vi "xcorr_packet bkp energy.vi"(0 "x":u32, 1 "y":u32, 2 "trigger":bool, 3 "normalization":u16) -> (8 "out":u64, 9 "valid":bool)   [LabVIEW 2017]
uses:
  <vilib>/rvi/FXPMathLib/FxpDiv/subVIs/nifxpmath_Div_SimConfig.ctl
  <vilib>/rvi/FXPMathLib/FxpDiv/simVIs/DllFxpDivTemp_sub.vi
  <vilib>/rvi/FXPMathLib/basic elements/FxpDiscreteDelay/XNode/nifxpmath_DiscreteDelay.xnode
  <vilib>/rvi/FXPMathLib/FxpMul/XNode/nifxpmath_Multiplier.xnode
  <vilib>/rvi/FXPMathLib/FxpDiv/XNode/nifxpmath_Div.xnode
  <vilib>/rvi/FXPMathLib/sim/FxpSim.dll
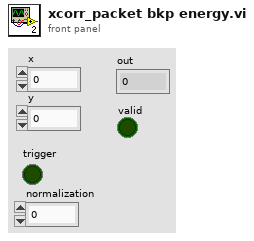
[diagram p1: front panel]
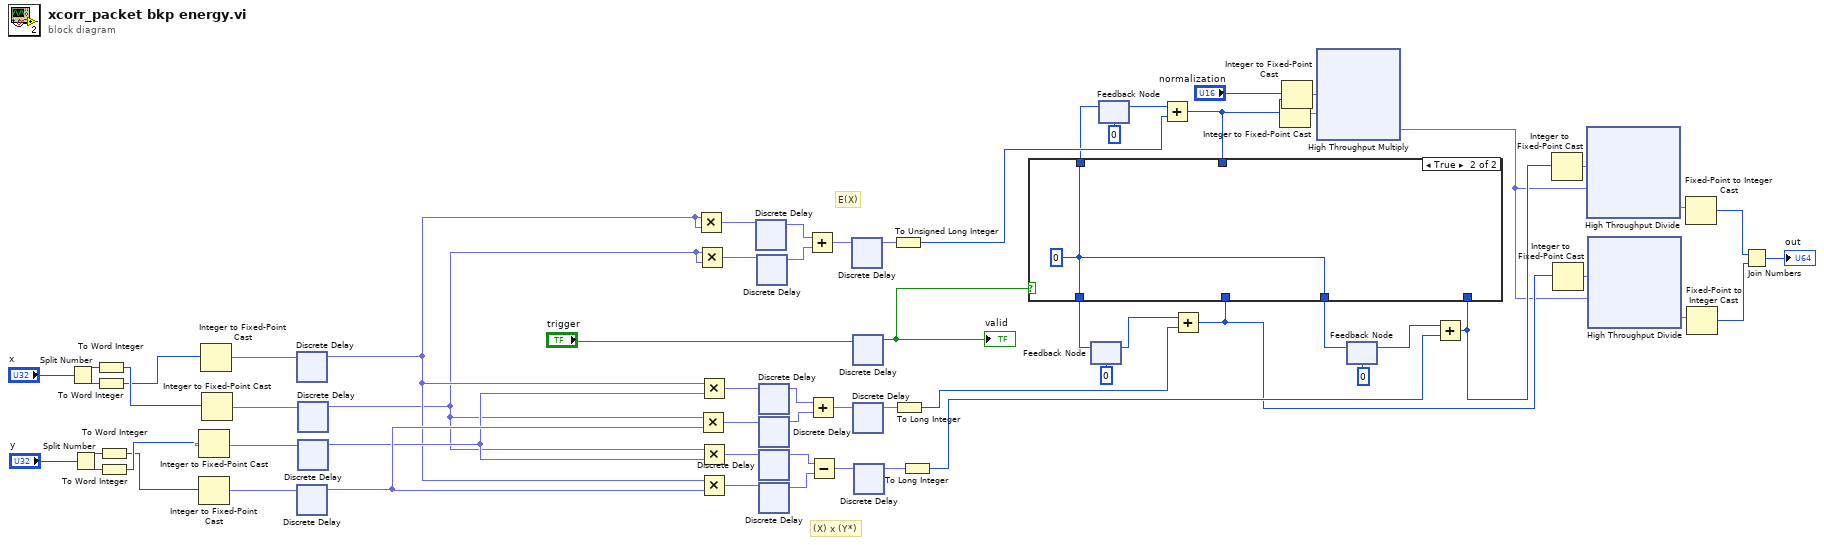
[diagram p0: block diagram]
diagram:
  # "E(X)"
  # "(X) x (Y*)"
  n1 = Split Number(x="x") -> (hi(x)=w55:u16, lo(x)=w56:u16)
  n2 = Split Number(x="y") -> (hi(x)=w57:u16, lo(x)=w58:u16)
  n3 = To Word Integer(number=w55) -> (16bit integer=w29:i16)
  n4 = To Word Integer(number=w56) -> (16bit integer=w28:i16)
  n5 = To Word Integer(number=w57) -> (16bit integer=w26:i16)
  n6 = To Word Integer(number=w58) -> (16bit integer=w27:i16)
  n7 = Integer to Fixed-Point Cast(integer=w27) -> (fixed-point=w38:fxp<+/-,16,16>)  [unwired: 1 in]
  n8 = Integer to Fixed-Point Cast(integer=w26) -> (fixed-point=w40:fxp<+/-,16,16>)  [unwired: 1 in]
  n9 = Integer to Fixed-Point Cast(integer=w28) -> (fixed-point=w36:fxp<+/-,16,16>)  [unwired: 1 in]
  n10 = Integer to Fixed-Point Cast(integer=w29) -> (fixed-point=w37:fxp<+/-,16,16>)  [unwired: 1 in]
  n11 = xnode "Discrete Delay"("D"=w36) -> ("Q"=w24:fxp<+/-,16,16>)
  n12 = xnode "Discrete Delay"("D"=w40) -> ("Q"=w39:fxp<+/-,16,16>)
  n13 = xnode "Discrete Delay"("D"=w37) -> ("Q"=w22:fxp<+/-,16,16>)
  n14 = xnode "Discrete Delay"("D"=w38) -> ("Q"=w34:fxp<+/-,16,16>)
  n15 = Multiply(x=w24, y=w24) -> (x*y=w25:fxp<+/-,32,32>)
  n16 = Multiply(x=w22, y=w22) -> (x*y=w23:fxp<+/-,32,32>)
  n17 = Multiply(x=w22, y=w39) -> (x*y=w46:fxp<+/-,32,32>)
  n18 = Multiply(x=w24, y=w34) -> (x*y=w45:fxp<+/-,32,32>)
  n19 = Multiply(x=w22, y=w34) -> (x*y=w47:fxp<+/-,32,32>)
  n20 = Multiply(x=w24, y=w39) -> (x*y=w48:fxp<+/-,32,32>)
  n21 = xnode "Discrete Delay"("D"=w25) -> ("Q"=w19:fxp<+/-,32,32>)
  n22 = xnode "Discrete Delay"("D"=w23) -> ("Q"=w18:fxp<+/-,32,32>)
  n23 = xnode "Discrete Delay"("D"=w45) -> ("Q"=w41:fxp<+/-,32,32>)
  n24 = xnode "Discrete Delay"("D"=w46) -> ("Q"=w42:fxp<+/-,32,32>)
  n25 = xnode "Discrete Delay"("D"=w47) -> ("Q"=w43:fxp<+/-,32,32>)
  n26 = xnode "Discrete Delay"("D"=w48) -> ("Q"=w44:fxp<+/-,32,32>)
  n27 = Add(x=w19, y=w18) -> (x+y=w20:fxp<+/-,33,33>)
  n28 = Add(x=w41, y=w42) -> (x+y=w51:fxp<+/-,33,33>)
  n29 = Subtract(x=w43, y=w44) -> (x-y=w50:fxp<+/-,32,32>)
  n30 = xnode "Discrete Delay"("D"=w20) -> ("Q"=w21:fxp<+/-,33,33>)
  n31 = xnode "Discrete Delay"("D"="trigger") -> ("Q"=w52:bool)
  "valid" <- w52
  n32 = xnode "Discrete Delay"("D"=w51) -> ("Q"=w35:fxp<+/-,33,33>)
  n33 = xnode "Discrete Delay"("D"=w50) -> ("Q"=w49:fxp<+/-,32,32>)
  n34 = To Unsigned Long Integer(number=w21) -> (unsigned 32bit integer=w15:u32)
  n35 = To Long Integer(number=w35) -> (32bit integer=w53:i32)
  n36 = To Long Integer(number=w49) -> (32bit integer=w54:i32)
  n37 = feedback #1(0) -> (w61:i32)
  n38 = feedback #2(0) -> (w16:u32)
  n39 = Add(x=w16, y=w15) -> (x+y=w2:u32)
  n40 = Add(x=w61, y=w53) -> (x+y=w8:i32)
  n41 = Integer to Fixed-Point Cast(integer=w2) -> (fixed-point=w3:fxp<+,32,32>)  [unwired: 1 in]
  n42 = Integer to Fixed-Point Cast(integer="normalization") -> (fixed-point=w4:fxp<+,16,16>)  [unwired: 1 in]
  n43 = xnode ("High Throughput Multiply")("x"=w4, "y"=w3) -> ("x*y"=w1:fxp<+,48,48>)
  n44 = feedback #3(0) -> (w31:i32)
  n45 = Add(x=w31, y=w54) -> (x+y=w9:i32)
  n46 = case shown="True" w52 {
    tunnel: [w67 w68] -> w32
    tunnel: [w66 w68] -> w30
    tunnel: w8 -> [w66 _]
    tunnel: w9 -> [w67 _]
    tunnel: [w65 w68] -> w14
    tunnel: w2 -> [w65 _]
    frame False {
    }
    frame True {
      w68 = 0
    }
  }
  n47 = feedback-in #1(w30) -> ()
  n48 = feedback-in #2(w14) -> ()
  n49 = feedback-in #3(w32) -> ()
  n50 = Integer to Fixed-Point Cast(integer=w9) -> (fixed-point=w10:fxp<+/-,32,32>)  [unwired: 1 in]
  n51 = Integer to Fixed-Point Cast(integer=w8) -> (fixed-point=w13:fxp<+/-,32,32>)  [unwired: 1 in]
  n52 = xnode "High Throughput Divide"("x"=w10, "y"=w1) -> ("x/y"=w11:fxp<+/-,32,32>)
  n53 = xnode "High Throughput Divide"("x"=w13, "y"=w1) -> ("x/y"=w12:fxp<+/-,32,32>)
  n54 = Fixed-Point to Integer Cast(1:w11) -> (0:w6:i32)
  n55 = Fixed-Point to Integer Cast(1:w12) -> (0:w7:i32)
  n56 = Join Numbers(hi=w6, lo=w7) -> ((hi.lo)=→"out":u64)
